vi "Create I2C object.vi"(10 "Position":u32, 11 "MTS I2C Test in":refnum<class "MTS I2C Test.lvclass">) -> (0 "error out":errorcluster, 3 "NI-8452 out":refnum<class "NI-8452.lvclass">)   [LabVIEW 2015, in "MTS I2C Test.lvclass"]
doc: "Creates and returns an NI-8452 device object."
uses:
  MTS I2C Test.lvclass
  Classes/Instruments/I2C Device/NI-8452/NI-8452.lvclass
  Classes/Instruments/I2C Device/I2C Device/Settings/Class Settings -- Cluster.ctl
  Classes/Test Recipe/Class/Test Recipe.lvclass
  Classes/Application/Class/Application.lvclass
  Test Class/Test Class.lvclass
  <vilib>/Cree, Inc/Cree Test Framework/Classes/Base Objects/Base Class/Base Class/Base Class.lvclass
  Classes/Instruments/I2C Device/I2C Device/Class/I2C Device.lvclass
  Classes/Instruments/I2C Device/I2C Device/Settings/I2C Device Settings.lvclass
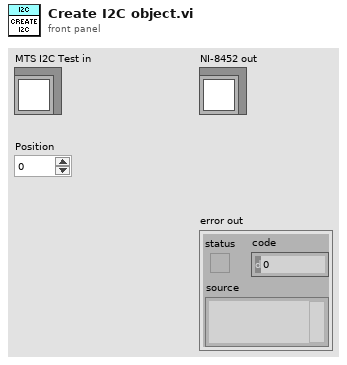
[diagram p1: front panel]
types:
  T1 = typedef "I2C Device.lvlib/I2C Device Settings.lvclass/Class Settings -- Cluster.ctl" = cluster{"ACK Timeout":u16, "Clockrate kHz":u16, "Address":u16, "DIO Direction Map":u8, "I/O Voltage Level":enum16{"3.3V", "2.5V", "1.8V", "1.5V", "1.2V"}, "I²C Pullup Enable":bool, "Number of Retries":u32, "I2C Type":enum16{"Master", "Slave"}}
  T2 = typedef "Application.lvlib/App Properties.lvclass/Class Properties -- Cluster.ctl" = cluster{"UUT Info":T3[], "Test Information":refnum<vi>, "Test Complete Event":refnum<user-event>, "Shop Floor System":refnum<class "Shop Floor System.lvclass">, "Gold Board":refnum<class "Golden Board.lvclass">, "Test Recipe":refnum<class "Test Recipe.lvclass">, "Instruments":refnum<class "Base Class.lvclass">[], "Mode":T4, "Test Results":cluster{"Pass":bool[], "Fail Codes":string[]}}
  T3 = typedef "Application.lvlib/App Properties.lvclass/UUT Reference -- Cluster.ctl" = cluster{"Serial Number Reference":refnum<vi>, "Status Message Reference":refnum<vi>}
  T4 = typedef "Application.lvlib/Application.lvclass/Op Mode -- Enum.ctl" = u16
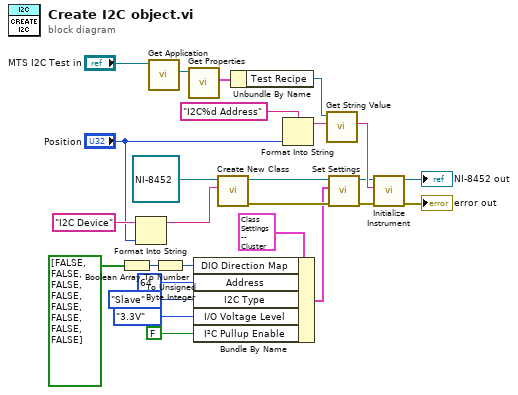
[diagram p0: block diagram]
diagram:
  n1 = Boolean Array To Number(Boolean array=bool[] [FALSE, FALSE, FALSE, FALSE, FALSE, FALSE, FALSE, FALSE]) -> (number=w15:u32)
  n2 = Format Into String(initial string="I2C Device" ("Name"), "Position") -> (resulting string=w2:string)  [unwired: 2 in, 1 out]
  n3 = call "Get Application.vi"("Test Class in"="MTS I2C Test in") -> ("Application.lvlib:Application.lvclass"=w9:refnum<class "Application.lvclass">)  [unwired: 9 in, 1 out]
  n4 = To Unsigned Byte Integer(number=w15) -> (unsigned 8bit integer=w14:u8)
  n5 = call "Get Properties.vi"("Acrobat Template in"=w9) -> ("Class Properties"=w8:T2)  [unwired: 8 in, 2 out]
  n6 = Bundle By Name(cluster=T1 {"ACK Timeout"=30000, "Clockrate kHz"=100, "Address"=64, "DIO Direction Map"=0, "I/O Voltage Level"=enum."3.3V", "I²C Pullup Enable"=FALSE, "Number of Retries"=3, "I2C Type"=enum."Master"} ("Class Settings"), "DIO Direction Map"=w14, "Address"=u16 64, "I2C Type"=enum16{"Master", "Slave"}."Slave", "I/O Voltage Level"=enum16{"3.3V", "2.5V", "1.8V", "1.5V", "1.2V"}."3.3V", "I²C Pullup Enable"=FALSE) -> (w17:T1)
  n7 = call <vilib>:"Create New Class.vi"("Name"=w2, "Base Class in"=refnum<class "NI-8452.lvclass"> refnum ("I2C Device.lvlib:NI-8452.lvclass")) -> ("error out"=w19:errorcluster, "Base Class out"=w20:refnum<class "NI-8452.lvclass">)  [unwired: 8 in]
  n8 = Unbundle By Name(w8) -> ("Test Recipe"=w10:refnum<class "Test Recipe.lvclass">)
  n9 = Format Into String(format string="I2C%d Address" ("Name"), "Position") -> (resulting string=w7:string)  [unwired: 2 in, 1 out]
  n10 = call "Get String Value.vi"("Name"=w7, "Test Recipe in"=w10) -> ("Value"=w26:string)  [unwired: 7 in, 2 out]
  n11 = call "Set Settings.vi"("error in (no error)"=w19, "Class Settings"=w17, "Acrobat Template in"=w20) -> ("error out"=w12:errorcluster, "Acrobat Template out"=w13:refnum<class "NI-8452.lvclass">)  [unwired: 7 in]
  n12 = call-dynamic "Initialize Instrument.vi"("error in (no error)"=w12, "Instrument Address"=w26, "Acrobat Template in"=w13) -> ("error out"=→"error out":errorcluster, "Acrobat Template out"=→"NI-8452 out":refnum<class "NI-8452.lvclass">)  [unwired: 7 in]
